vi "GE 5565PIORC.Registers.Write (U8).vi"(7 "Address Space":T1=11 items=["VXI/VME A16"=1, "VXI/VME A24"=2, "VXI/VME A32"=3, "VXI/VME A64"=4, "PXI Memory Allocations"=9, "PXI Configuration"=10, "PXI BAR0"=11, "PXI BAR1"=12, "PXI BAR2"=13, "PXI BAR3"=14, "PXI BAR4"=15, "PXI BAR5"=16], 8 "error in (no error)":errorcluster, 9 "Value":u8, 10 "Offset":u32, 11 "GE 5565PIORC in":refnum<class "GE 5565PIORC.lvclass">) -> (0 "error out":errorcluster, 3 "GE 5565PIORC out":refnum<class "GE 5565PIORC.lvclass">)   [LabVIEW 2016, in "GE 5565PIORC.lvclass"]
uses:
  GE 5565PIORC.lvclass
  <vilib>/Instr/_visa.llb/VISA Register Access Address Space.ctl
  GE 5565PIORC.lvclass/GE 5565PIORC.ctl
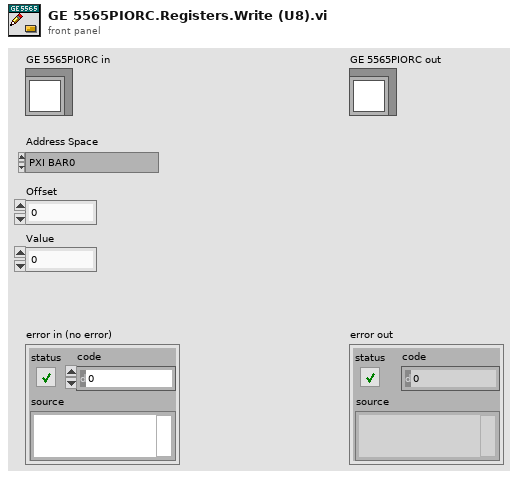
[diagram p1: front panel]
types:
  T1 = typedef "VISA Register Access Address Space.ctl" = u16
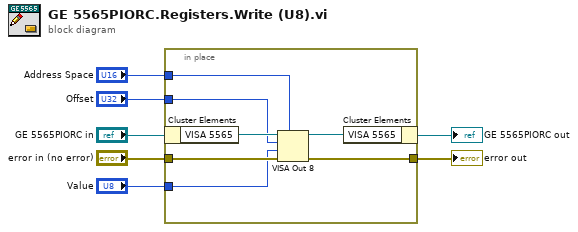
[diagram p0: block diagram]
diagram:
  n1 = in-place {
    in-place-border: "error in (no error)" -> [w12]
    in-place-border: [w11] -> w3
    in-place-border: "Address Space" -> [w10]
    in-place-border: "Offset" -> [w9]
    in-place-border: "Value" -> [w8]
    n2 = in-place-cluster #1("GE 5565PIORC in") -> ("VISA 5565"=w14:refnum<visa-resource-name>)
    n3 = VISA Out 8(7:w10, 8:w12, 9:w8, 10:w9, 11:w14) -> (0:w11:errorcluster, 3:w13:refnum<visa-resource-name>)
    n4 = in-place-cluster #1("VISA 5565"=w13) -> (→"GE 5565PIORC out":refnum<class "GE 5565PIORC.lvclass">)
  }
  "error out" <- w3
